vi "KeyenceCVX.Main.Close.vi"(8 "error in":errorcluster, 11 "Data in":T1 {"Status"."TriggerNo" items=["1"=1, "2"=2, "3"=3, "4"=4, "ALL"=5]}) -> (0 "error out":errorcluster, 3 "Data out":T1 {"Status"."TriggerNo" items=["1"=1, "2"=2, "3"=3, "4"=4, "ALL"=5]})   [LabVIEW 2016]
uses:
  KeyenceCVX.Data.ctl
  KeyenceCVX.Data.Status.ctl
  KeyenceCVX.Data.Status.State.ctl
  private/controls/TriggerNo.ctl
  private/controls/RunMode.ctl
  KeyenceCVX.Data.Sets.ctl
  KeyenceCVX.CodeDetails.ctl
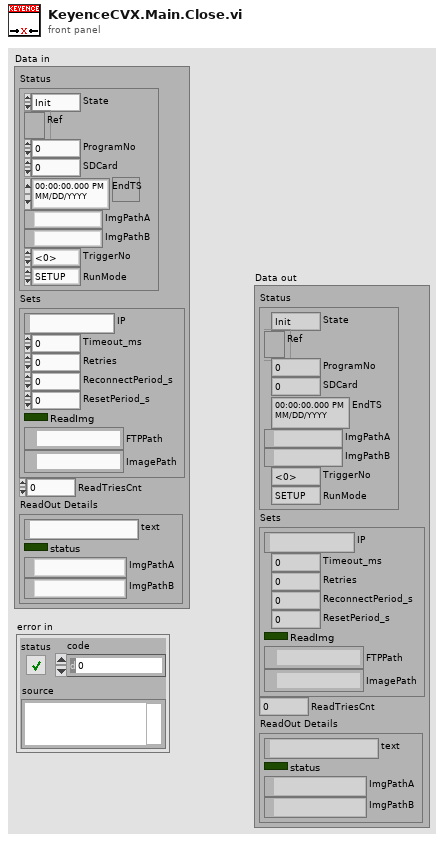
[diagram p1: front panel]
types:
  T1 = typedef "KeyenceCVX.Data.ctl" = cluster{"Status":T2, "Sets":T6, "ReadTriesCnt":u8, "ReadOut Details":T7}
  T2 = typedef "KeyenceCVX.Data.Status.ctl" = cluster{"State":T3, "Ref":refnum<k5>, "ProgramNo":u16, "SDCard":u8, "EndTS":timestamp, "ImgPathA":path, "ImgPathB":path, "TriggerNo":T4, "RunMode":T5}
  T3 = typedef "KeyenceCVX.Data.Status.State.ctl" = enum16{"Init", "Idle", "Scan", "Reset", "ScanAck", "ChangeProgram"}
  T4 = typedef "TriggerNo.ctl" = u8
  T5 = typedef "RunMode.ctl" = enum16{"SETUP", "RUN"}
  T6 = typedef "KeyenceCVX.Data.Sets.ctl" = cluster{"IP":string, "Timeout_ms":i32, "Retries":i32, "ReconnectPeriod_s":i32, "ResetPeriod_s":i32, "ReadImg":bool, "FTPPath":path, "ImagePath":path}
  T7 = typedef "KeyenceCVX.CodeDetails.ctl" = cluster{"text":string, "status":bool, "ImgPathA":path, "ImgPathB":path}
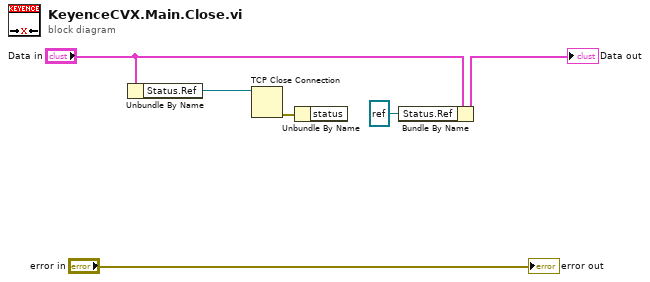
[diagram p0: block diagram]
diagram:
  n1 = Unbundle By Name("Data in") -> ("Status.Ref"=w4:refnum<k5>)
  n2 = TCP Close Connection(connection ID=w4) -> (error out=w5:errorcluster)  [unwired: 2 in, 1 out]
  n3 = Unbundle By Name(w5) -> ()  [unwired: 1 out]
  n4 = Bundle By Name(cluster="Data in", "Status.Ref"=refnum<k5> refnum) -> (→"Data out":T1)
  "error out" <- "error in"
